vi "DetectAndOpenStages.vi"(8 "error in (no error)":errorcluster, 11 "Config In":T1) -> (0 "error out":errorcluster, 3 "Config Out":T1)   [LabVIEW 2019]
uses:
  Settings/Settings.ctl
  Support/Hardware Configuration.ctl
  Support/Camera Configuration.ctl
  E:/DevHardSoftware/MMicroscopy/HardwareAdapter/Camera/Dependencies/PVCamNET.dll
  Camera/Dependencies/PVCamNET.dll
  <vilib>/userdefined/High Color/IMAQdx.ctl
  Logging/Logging Configuration.ctl
  controls/UI Configuration.ctl
  Dependencies/Madlib.dll
  Dependencies/MicroDrive.dll
  Dependencies/TIRF-Lock.dll
  Logging/Logging.lvlib
  Settings/Settings.lvlib
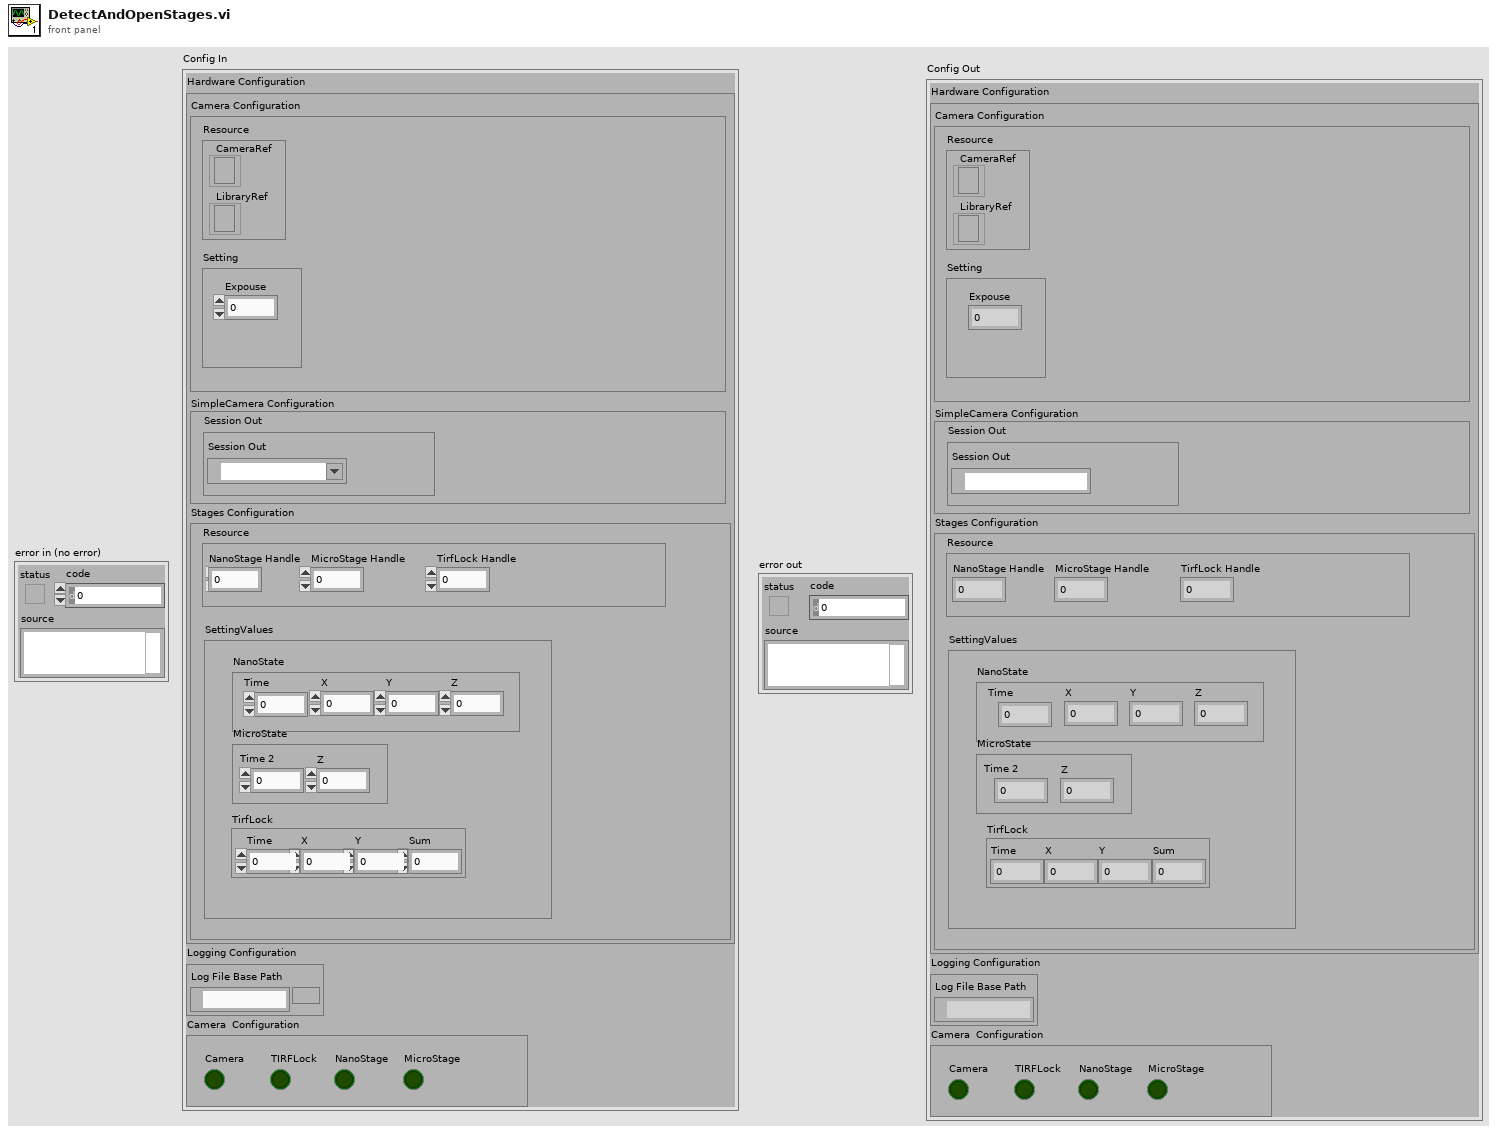
[diagram p1: front panel]
types:
  T1 = typedef "Settings.lvlib/Settings.ctl" = cluster{"Hardware Configuration":T2, "Logging Configuration":T5, "UI Configuration":T6}
  T2 = typedef "Hardware Configuration.ctl" = cluster{"Camera Configuration":T3, "SimpleCamera Configuration":cluster{"Resource":cluster{"Session Out":T4}}, "Stages Configuration":cluster{"Resource":cluster{"NanoStage Handle":i32, "MicroStage Handle":i32, "TirfLock Handle":i32}, "SettingValues":cluster{"NanoState":cluster{"Time":dbl, "X":dbl, "Y":dbl, "Z":dbl}, "MicroState":cluster{"Time 2":dbl, "Z":dbl}, "TirfLock":cluster{"Time":dbl, "X":dbl, "Y":dbl, "Sum":dbl}}}}
  T3 = typedef "Camera Configuration.ctl" = cluster{"Resource":cluster{"CameraRef":refnum<k24>, "LibraryRef":refnum<k24>}, "Setting":cluster{"Expouse":dbl}}
  T4 = typedef "IMAQdx.ctl" = refnum<k21>
  T5 = typedef "Logging.lvlib/Logging Configuration.ctl" = cluster{"Log File Base Path":path}
  T6 = typedef "UI Configuration.ctl" = cluster{"Camera":bool, "NanoStage":bool, "MicroStage":bool, "TIRFLock":bool}
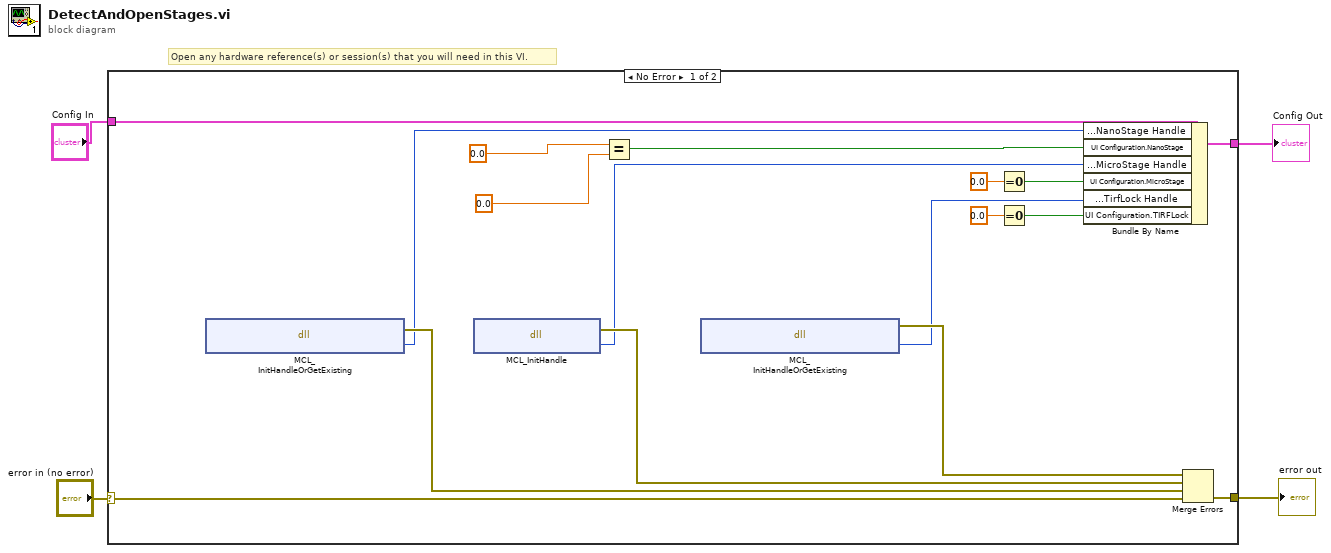
[diagram p0: block diagram]
diagram:
  # "Open any hardware reference(s) or session(s) that you will need in this VI."
  n1 = case shown="No Error" "error in (no error)" {
    selector: "error in (no error)" -> [w18 w22]
    tunnel: [w21 w22] -> w3
    tunnel: "Config In" -> [w20 w23]
    tunnel: [w19 w23] -> w1
    frame No Error {
      n2 = dll-call lib="E:/DevHardSoftware/MMicroscopy/HardwareAdapter/Stages/Dependencies/Madlib.dll" fn="MCL_InitHandleOrGetExisting"() -> (error out=w11:errorcluster, "return type"=w9:i32)  [unwired: 3 in, 1 out]
      n3 = dll-call lib="E:/DevHardSoftware/MMicroscopy/HardwareAdapter/Stages/Dependencies/MicroDrive.dll" fn="MCL_InitHandle"() -> (error out=w17:errorcluster, "return type"=w13:i32)  [unwired: 3 in, 1 out]
      n4 = Equal?(x=0.0, y=0.0) -> (x = y?=w8:bool)
      n5 = dll-call lib="E:/DevHardSoftware/MMicroscopy/HardwareAdapter/Stages/Dependencies/TIRF-Lock.dll" fn="MCL_InitHandleOrGetExisting" label="TIRF handle"() -> (error out=w16:errorcluster, "handle"=w15:i32)  [unwired: 3 in, 1 out]
      n6 = Equal To 0?(x=0.0) -> (x = 0?=w12:bool)
      n7 = Equal To 0?(x=0.0) -> (x = 0?=w14:bool)
      n8 = Bundle By Name(cluster=w20, "Hardware Configuration.Stages Configuration.Resource.NanoStage Handle"=w9, "UI Configuration.NanoStage"=w8, "Hardware Configuration.Stages Configuration.Resource.MicroStage Handle"=w13, "UI Configuration.MicroStage"=w12, "Hardware Configuration.Stages Configuration.Resource.TirfLock Handle"=w15, "UI Configuration.TIRFLock"=w14) -> (w19:T1)
      n9 = Merge Errors(w16, w17, w11, w18) -> (w21:errorcluster)
    }
    frame Error {
    }
  }
  "error out" <- w3
  "Config Out" <- w1
